vi "Get Key Value (Boolean).vi"(5 "Key name":string, 6 "Default value":bool, 7 "Section name":string, 8 "error in (no error)":errorcluster, 11 "Carya Config in":refnum<class "Carya Config.lvclass">) -> (0 "error out":errorcluster, 1 "Found?":bool, 2 "Value":bool, 3 "Carya Config out":refnum<class "Carya Config.lvclass">)   [LabVIEW 2013, in "Carya Config.lvclass"]
doc: "Copyright 2018, Carya Automatisering, Wiebe Walstra."
uses:
  Carya Config.lvclass
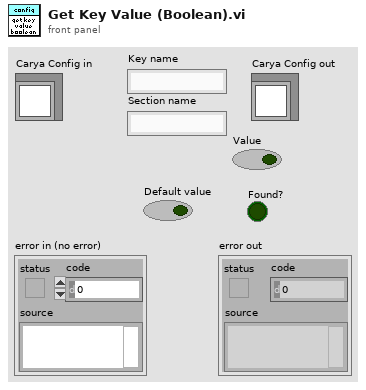
[diagram p1: front panel]
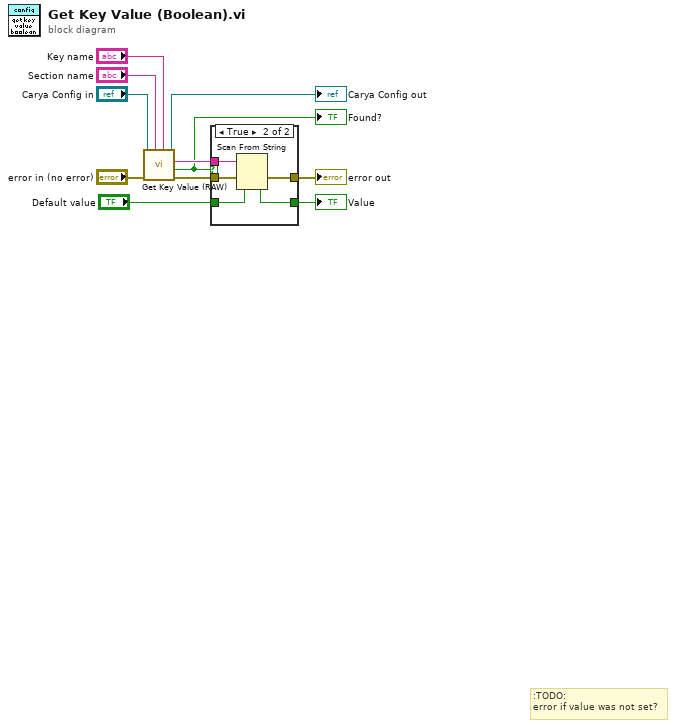
[diagram p0: block diagram]
diagram:
  # ":TODO:\nerror if value was not set?"
  n1 = call-dynamic "Get Key Value (RAW).vi"("Key name"="Key name", "Section name"="Section name", "error in (no error)"="error in (no error)", "Carya Config in"="Carya Config in") -> ("error out"=w10:errorcluster, "Found?"=w2:bool, "Value"=w4:string, "Carya Config out"=→"Carya Config out":refnum<class "Carya Config.lvclass">)  [unwired: 4 in]
  "Found?" <- w2
  n2 = case shown="True" w2 {
    tunnel: w10 -> [w12 w18]
    tunnel: [w12 w17] -> w5
    tunnel: w4 -> [_ w16]
    tunnel: "Default value" -> [w13 w15]
    tunnel: [w13 w14] -> w1
    frame False {
    }
    frame True {
      n3 = Scan From String(input string=w16, error in=w18, default 1=w15) -> (error out=w17:errorcluster, output 1=w14:bool)  [unwired: 2 in, 2 out]
    }
  }
  "error out" <- w5
  "Value" <- w1
